vi "GCSArray_regex_matches.vi"(0 "GCSArray input string":string, 1 "Selector":T2, 2 "Range":T1, 5 "error in (no error)":errorcluster) -> (14 "Matches":string[](array[string]), 19 "error out":errorcluster)   [LabVIEW 2026]
doc: "Decomposes a human readable GCSArray datastream (Input string) into subpieces (Matches). The searchable area in Input string is limited with the Range control values. The value of Selector specifies, what type of information will be transferred to Matches."
uses:
  GCSArray_regex_selector.ctl
  GCSArray_regex_range.ctl
  <vilib>/regexp/Match Regular Expression.xnode
panel:
  # "Select parts ('Selector') of a GCSArray ('Input string')\nand return all found entries ('Matches')."
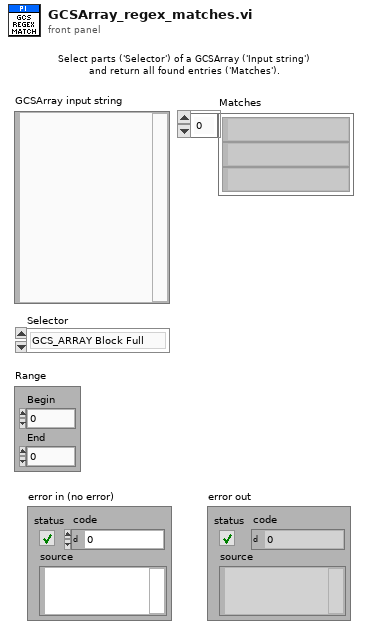
[diagram p1: front panel]
types:
  T1 = typedef "GCSArray_regex_range.ctl" = cluster{"Begin":i32, "End":i32}
  T2 = typedef "GCSArray_regex_selector.ctl" = enum16{"GCS_ARRAY Block Full", "GCS_ARRAY Block ID", "GCS_ARRAY Block Header", "GCS_ARRAY Block Data", "GCS_ARRAY Identifier", "GCS_ARRAY Remark", "GCS_ARRAY Version", "GCS_ARRAY Dimension", "GCS_ARRAY Type", "GCS_ARRAY Separator", "GCS_ARRAY NData", "GCS_ARRAY NData%", "GCS_ARRAY NData% Keyword", "GCS_ARRAY Name%", "GCS_ARRAY Name% Keyword", "GCS_ARRAY Start%", "GCS_ARRAY Start% Keyword", "GCS_ARRAY End%", "GCS_ARRAY End% Keyword", "GCS_ARRAY Delta%", "GCS_ARRAY Delta% Keword", "GCS_ARRAY Sample Time", "GCS_ARRAY Unit of transmitted value%", "GCS_ARRAY Trans_Unit% Keyword", "GCS_ARRAY Trans_Unit% = RAW Keyword", "GCS_ARRAY Unit of displayed value%", "GCS_ARRAY Disp_Unit% Keyword", "GCS_ARRAY Nominator%", "GCS_ARRAY Ratio_Nom% Keyword", "GCS_ARRAY Denominator%", "GCS_ARRAY Ratio_Denom% Keyword", "GCS_ARRAY End of Header", "GCS_ARRAY Empty line of Header"}
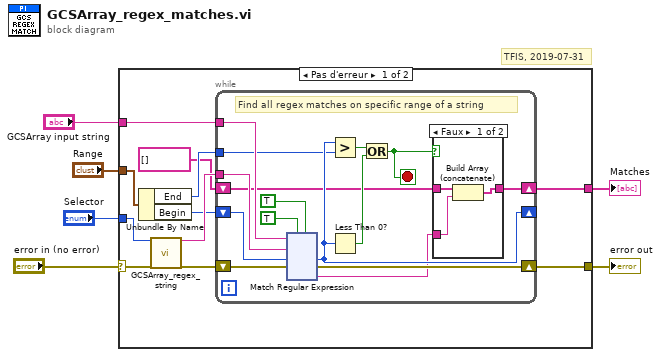
[diagram p0: block diagram]
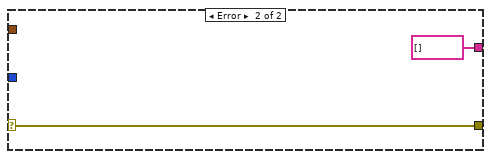
[diagram p3: hidden frame]
diagram:
  # "TFIS, 2019-07-31"
  n1 = case shown="Pas d'erreur" "error in (no error)" {
    selector: "error in (no error)" -> [w13 w157]
    tunnel: [w17 w157] -> w5
    tunnel: "GCSArray input string" -> [w16 _]
    tunnel: "Selector" -> [w15 _]
    tunnel: "Range" -> [w11 _]
    tunnel: [w9 string[] []] -> w1
    frame No Error {
      n2 = Unbundle By Name(w11) -> ("End"=w8:i32, "Begin"=w10:i32)
      n3 = call "GCSArray_regex_string.vi"("Selector"=w15, "error in (no error)"=w13) -> ("Regex string"=w14:string, "error out"=w12:errorcluster)  [unwired: 16 out]
      n4 = while {
        shift-right: [w30] -> w17
        shift-left: w12 -> [w23]
        shift-right: [w28] -> _
        shift-left: w10 -> [w29]
        tunnel: w16 -> [w25]
        tunnel: w14 -> [w24]
        tunnel: w8 -> [w21]
        shift-right: [w19] -> w9
        shift-left: string[] [] ("Array") -> [w20]
        stop <- w18 stop-if-true
        # "Find all regex matches on specific range of a string"
        n5 = xnode "Match Regular Expression"("chaîne en entrée"=w25, "expression régulière"=w24, "offset (0)"=w29, "entrée d'erreur"=w23, "ignorer la casse ? (F)"=TRUE ("ignore case? (F)"), "multiligne ? (F)"=TRUE ("multiline? (F)")) -> ("offset après correspondance"=w28:i32, "sortie d'erreur"=w30:errorcluster, "correspondance partielle 1"=w22:string)  [unwired: 3 out]
        n6 = Greater?(x=w28, y=w21) -> (0:w27:bool)
        n7 = Less Than 0?(x=w28) -> (x < 0?=w26:bool)
        n8 = Or(x=w27, y=w26) -> (x .or. y?=w18:bool)
        n9 = case shown="Faux" w18 {
          tunnel: w20 -> [w34 w36]
          tunnel: w22 -> [w33 _]
          tunnel: [w35 w36] -> w19
          frame False {
            n10 = Build Array (concatenate)(w34, w33) -> (w35:string[])
          }
          frame True {
          }
        }
      }
    }
    frame Error {
    }
  }
  "error out" <- w5
  "Matches" <- w1
